vi "SeparaMemoriaStatusMotor.vi"(8 "error in":errorcluster) -> (0 "error out":errorcluster, 3 "Memorias":T1(array[cluster]))   [LabVIEW 2019]
uses:
  TelaConfig/Configuracao.Variaveis.vi
  VariaveisMedicao.vi
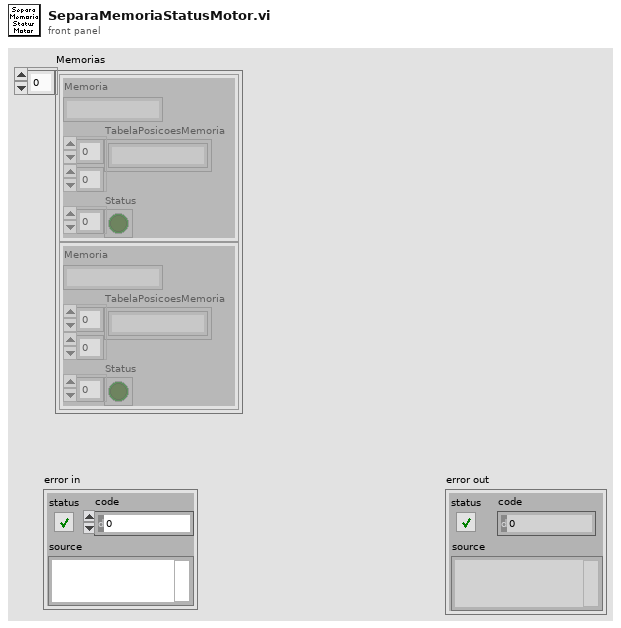
[diagram p1: front panel]
types:
  T1 = cluster{"Memoria":string, "TabelaPosicoesMemoria":string[][], "Status":bool[]}[]
  T2 = cluster{"Memoria":string, "TabelaPosicoesMemoria":string[][], "Status":bool[]}
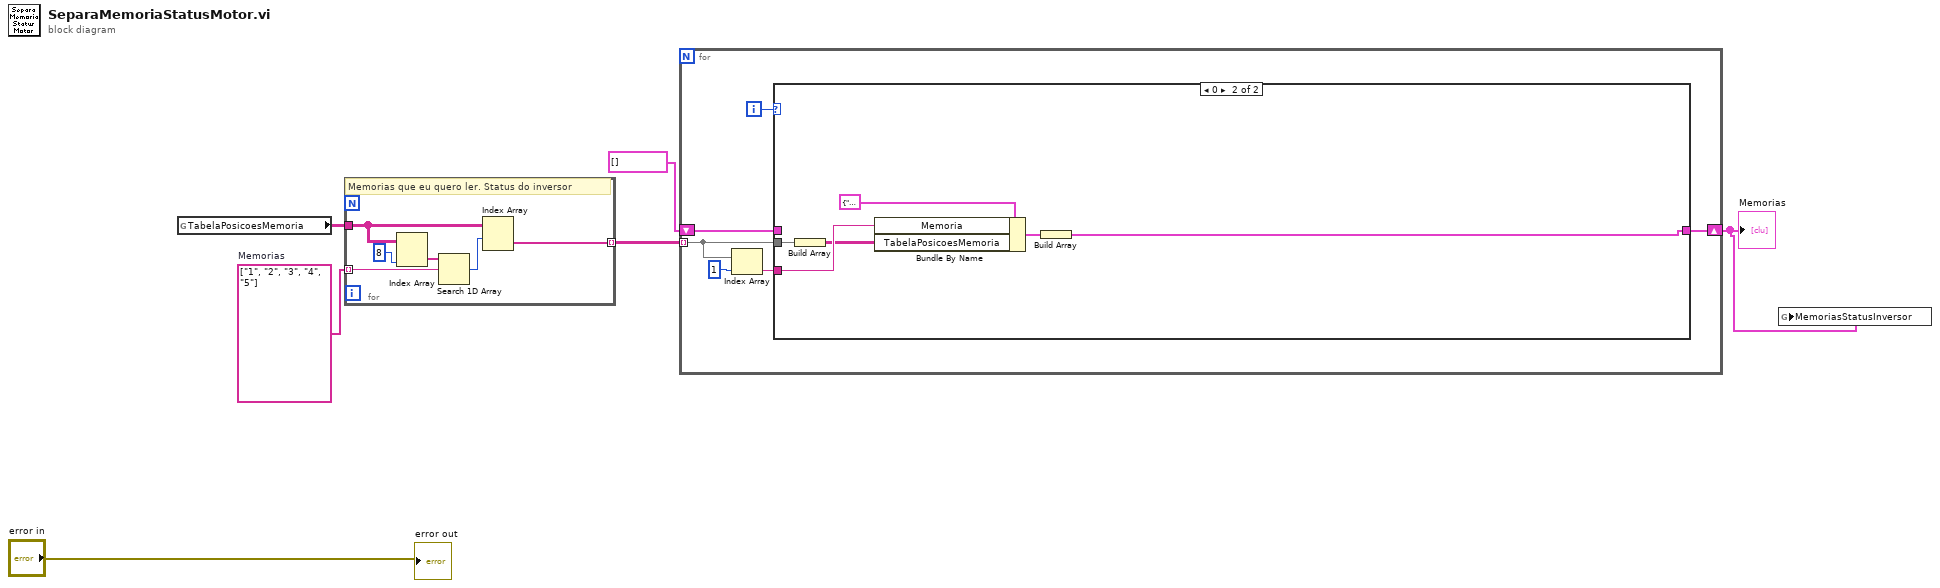
[diagram p0: block diagram]
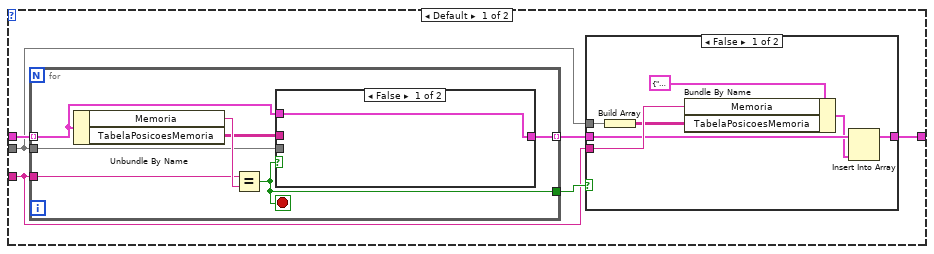
[diagram p2: hidden frame]
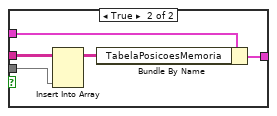
[diagram p4: hidden frame]
diagram:
  w6 = string[] ["1", "2", "3", "4", "5"]  # Memorias
  n1 = global read "Configuracao.Variaveis.vi" "TabelaPosicoesMemoria"() -> (w3:string[][])
  n2 = for {
    tunnel: w3 -> [w8]
    tunnel: w6 -> [w9] mode=indexing
    tunnel: [w7] -> w5 mode=indexing
    # "Memorias que eu quero ler. Status do inversor"
    n3 = Index Array(array=w8, index (col)=8 ("disabled index (col)")) -> (element=w10:string[])  [unwired: 1 in]
    n4 = Search 1D Array(1D array=w10, element=w9) -> (index of element=w12:i32)  [unwired: 1 in]
    n5 = Index Array(array=w8, index (row)=w12) -> (element=w7:string[])  [unwired: 1 in]
  }
  n6 = for {
    tunnel: w5 -> [w15] mode=indexing
    shift-right: [w14] -> w2
    shift-left: T1 [] ("Memorias") -> [w13]
    i -> [w17]
    n7 = Index Array(array=w15, index=1) -> (element=w16:string)
    n8 = case shown="0" w17 {
      tunnel: w16 -> [w20 w51]
      tunnel: w15 -> [w19 w50]
      tunnel: [w22 w47] -> w14
      tunnel: w13 -> [w24 _]
      frame Default {
        n9 = for {
          tunnel: w24 -> [w37] mode=indexing
          tunnel: w20 -> [w38]
          tunnel: w19 -> [w35]
          tunnel: [w34] -> w21 mode=indexing
          tunnel: [w33] -> w23
          stop <- w33 stop-if-true
          n10 = Unbundle By Name(w37) -> ("Memoria"=w39:string, "TabelaPosicoesMemoria"=w36:string[][])
          n11 = Equal?(x=w38, y=w39) -> (x = y?=w33:bool)
          n12 = case shown="False" w33 {
            tunnel: w37 -> [w40 w45]
            tunnel: w36 -> [_ w44]
            tunnel: w35 -> [_ w43]
            tunnel: [w40 w41] -> w34
            frame False {
            }
            frame True {
              n13 = Insert Into Array(array=w44, new element=w43) -> (w42:string[][])  [unwired: 2 in]
              n14 = Bundle By Name(cluster=w45, "TabelaPosicoesMemoria"=w42) -> (w41:T2)
            }
          }
        }
        n15 = case shown="False" w23 {
          tunnel: [w25 w32] -> w22
          tunnel: w21 -> [w27 w32]
          tunnel: w20 -> [w30 _]
          tunnel: w19 -> [w29 _]
          frame False {
            n16 = Build Array(w29) -> (w28:string[][])
            n17 = Bundle By Name(cluster=T2 {"Memoria"="", "TabelaPosicoesMemoria"=[], "Status"=[]} ("Cluster"), "Memoria"=w30, "TabelaPosicoesMemoria"=w28) -> (w26:T2)
            n18 = Insert Into Array(array=w27, new element=w26) -> (w25:T1)  [unwired: 1 in]
          }
          frame True {
          }
        }
      }
      frame 0 {
        n19 = Build Array(w50) -> (w49:string[][])
        n20 = Bundle By Name(cluster=T2 {"Memoria"="", "TabelaPosicoesMemoria"=[], "Status"=[]} ("Cluster"), "Memoria"=w51, "TabelaPosicoesMemoria"=w49) -> (w48:T2)
        n21 = Build Array(w48) -> (w47:T1)
      }
    }
  }
  "Memorias" <- w2
  n22 = global write "VariaveisMedicao.vi" "MemoriasStatusInversor"(w2) -> ()
  "error out" <- "error in"
